vi "Write Data.vi"(0 "Error Logger in":refnum<class "Error Logger.lvclass">, 7 "Error Data":T1, 11 "error in (no error)":errorcluster) -> (4 "Error Logger out":refnum<class "Error Logger.lvclass">, 15 "error out":errorcluster)   [LabVIEW 2014, in "Error Logger.lvclass"]
uses:
  Error Logger.lvclass
  Controls/Error Data.ctl
  Error Logger.lvclass/Error Logger.ctl
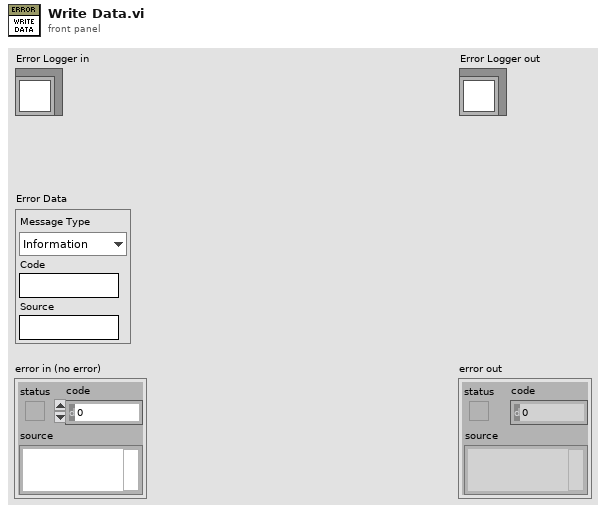
[diagram p1: front panel]
types:
  T1 = typedef "Error Logger.lvclass/Error Data.ctl" = cluster{"Message Type":enum16{"Information", "Warning", "Error"}, "Code":string, "Source":string}
  T2 = enum16{"open", "replace", "create", "open or create", "replace or create", "replace or create with confirmation"}
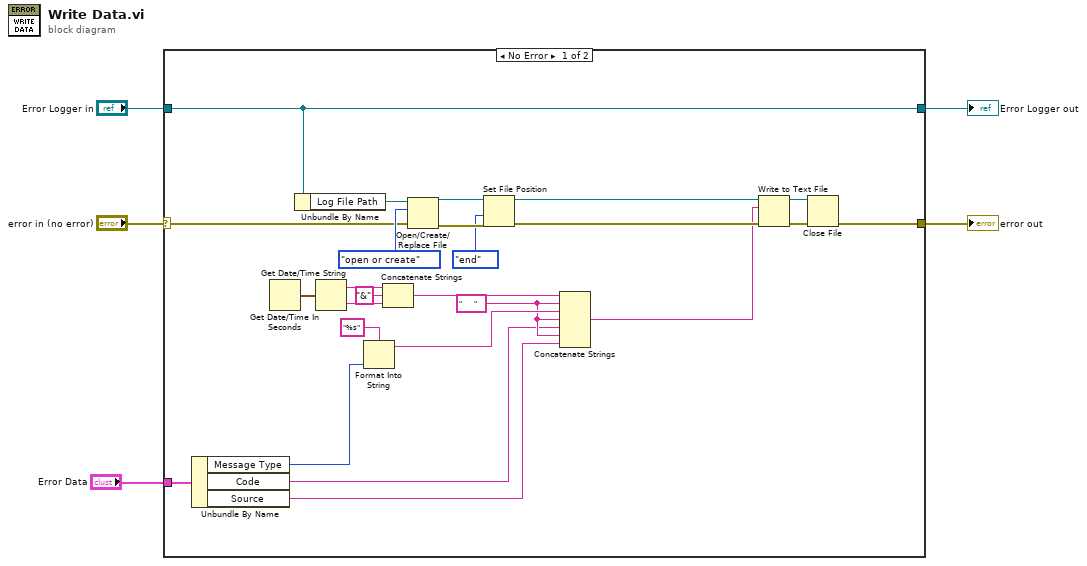
[diagram p0: block diagram]
diagram:
  n1 = case shown="No Error" "error in (no error)" {
    selector: "error in (no error)" -> [w20 w32]
    tunnel: [w12 w32] -> w4
    tunnel: [w22 w31] -> w2
    tunnel: "Error Logger in" -> [w22 w31]
    tunnel: "Error Data" -> [w9 _]
    frame No Error {
      w11 = "      " ("string")
      n2 = Unbundle By Name(w9) -> ("Message Type"=w8:enum16{"Information", "Warning", "Error"}, "Code"=w7:string, "Source"=w6:string)
      n3 = Get Date/Time In Seconds() -> (seconds since 1Jan1904=w19:timestamp)
      n4 = Unbundle By Name(w22) -> ("Log File Path"=w21:path)
      n5 = Get Date/Time String(seconds (now)=w19) -> (date string=w18:string, time string=w17:string)  [unwired: 2 in]
      n6 = Format Into String(format string="%s", w8) -> (resulting string=w13:string)  [unwired: 2 in, 1 out]
      n7 = Concatenate Strings(w18, "&" ("string"), w17) -> (w16:string)
      n8 = Open/Create/Replace File(file path (use dialog)=w21, error in=w20, operation (0:open)=T2."open or create") -> (refnum out=w29:refnum<file>, error out=w28:errorcluster)  [unwired: 3 in, 1 out]
      n9 = Set File Position(refnum=w29, from (0:start)=enum16{"start", "end", "current"}."end", error in=w28) -> (refnum out=w26:refnum<file>, error out=w25:errorcluster)  [unwired: 1 in]
      n10 = Concatenate Strings(w16, w11, w13, w11, w7, w11, w6) -> (w10:string)
      n11 = Write to Text File(file (use dialog)=w26, text=w10, error in=w25) -> (refnum out=w23:refnum<file>, error out=w24:errorcluster)  [unwired: 1 in, 1 out]
      n12 = Close File(refnum=w23, error in=w24) -> (error out=w12:errorcluster)  [unwired: 1 out]
    }
    frame Error {
    }
  }
  "error out" <- w4
  "Error Logger out" <- w2
